vi "Check Start or Stop.vi"(8 "error in (no error)":errorcluster, 9 "Target (All)":string, 10 "Log Group (All)":T1, 11 "GroupLoggingControl in":refnum<class "GroupLoggingControl.lvclass">) -> (0 "error out":errorcluster, 2 "Logging":bool, 3 "GroupLoggingControl out":refnum<class "GroupLoggingControl.lvclass">)   [LabVIEW 2020, in "VolatusGUIElements.lvlib" / "GroupLoggingControl.lvclass"]
uses:
  GroupLoggingControl.lvclass
  Log Group.ctl
  Log Group Status.ctl
  Command Info.ctl
  GroupLoggingControl.lvclass/GroupLoggingControl.ctl
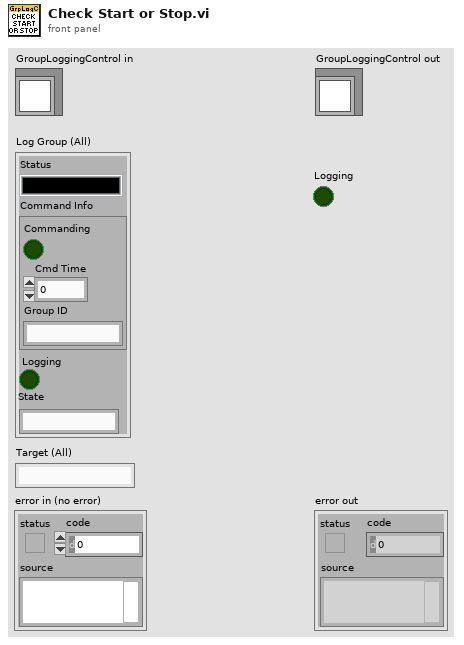
[diagram p1: front panel]
types:
  T1 = typedef "VolatusGUIElements.lvlib/GroupLoggingControl.lvclass/Log Group.ctl" = cluster{"Status":T2, "Command Info":T3, "Logging":bool, "State":string}
  T2 = typedef "VolatusGUIElements.lvlib/GroupLoggingControl.lvclass/Log Group Status.ctl" = cluster{"Group":string, "Group Color":u32, "Button":bool}
  T3 = typedef "VolatusGUIElements.lvlib/GroupLoggingControl.lvclass/Command Info.ctl" = cluster{"Commanding":bool, "Cmd Time":dbl, "Group ID":string}
  T4 = typedef "VolatusGUIElements.lvlib/GroupLoggingControl.lvclass/Target Info.ctl" = cluster{"Node":string, "Node Color":u32, "Groups":T1[]}
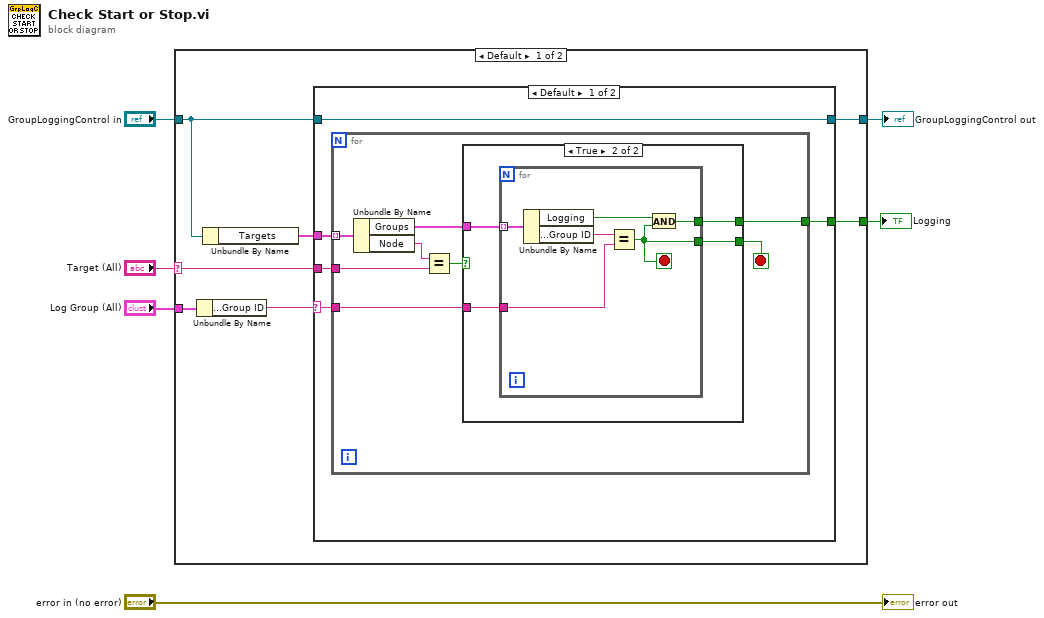
[diagram p0: block diagram]
diagram:
  n1 = case shown="Default" "Target (All)" {
    selector: "Target (All)" -> [w9 _]
    tunnel: "GroupLoggingControl in" -> [w12 w38]
    tunnel: "Log Group (All)" -> [w13 _]
    tunnel: [w8 w38] -> w2
    tunnel: [w7 _] -> w1
    frame Default {
      n2 = Unbundle By Name(w13) -> ("Command Info.Group ID"=w11:string)
      n3 = Unbundle By Name(w12) -> ("Targets"=w10:T4[])
      n4 = case shown="Default" w11 {
        selector: w11 -> [w15 _]
        tunnel: w12 -> [w18 w37]
        tunnel: w10 -> [w17 _]
        tunnel: w9 -> [w16 _]
        tunnel: [w18 w37] -> w8
        tunnel: [w14 _] -> w7
        frame Default {
          n5 = for {
            tunnel: w17 -> [w26] mode=indexing
            tunnel: w16 -> [w25]
            tunnel: w15 -> [w21]
            tunnel: [w20] -> w14
            stop <- w19 stop-if-true
            n6 = Unbundle By Name(w26) -> ("Groups"=w22:T1[], "Node"=w24:string)
            n7 = Equal?(x=w24, y=w25) -> (x = y?=w23:bool)
            n8 = case shown="True" w23 {
              tunnel: w22 -> [_ w30]
              tunnel: w21 -> [_ w29]
              tunnel: [_ w28] -> w20
              tunnel: [_ w27] -> w19
              frame False {
              }
              frame True {
                n9 = for {
                  tunnel: w30 -> [w36] mode=indexing
                  tunnel: w29 -> [w34]
                  tunnel: [w32] -> w28
                  tunnel: [w31] -> w27
                  stop <- w31 stop-if-true
                  n10 = Unbundle By Name(w36) -> ("Logging"=w33:bool, "Command Info.Group ID"=w35:string)
                  n11 = Equal?(x=w35, y=w34) -> (x = y?=w31:bool)
                  n12 = And(x=w33, y=w31) -> (x .and. y?=w32:bool)
                }
              }
            }
          }
        }
        frame "True" {
        }
      }
    }
    frame "" {
      # "All Targets"
    }
  }
  "GroupLoggingControl out" <- w2
  "Logging" <- w1
  "error out" <- "error in (no error)"
